vi "_Copy 1.vi"(0 "XRef":T5, 1 "State In":T1) -> (14 "Reply":T3, 15 "Fatal Error Out":T2, 16 "State Out":T1)   [LabVIEW 2014, in "JKISM++ DebugTool.xnode"]
uses:
  JKISM++ DebugTool.xnode
  <vilib>/XNodeSupport/XNodeXNodeRef.ctl
  _State 1.ctl
  <vilib>/XNodeSupport/XNodeStringArray.ctl
  <vilib>/XNodeSupport/XNodeString.ctl
  <vilib>/XNodeSupport/XNodeErrorCluster.ctl
  <vilib>/XNodeSupport/NI_XNodeSupport.lvlib
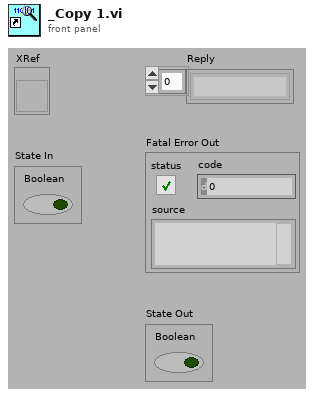
[diagram p1: front panel]
types:
  T1 = typedef "JKISM++ DebugTool.xnode/_State 1.ctl" = cluster{"Boolean":bool}
  T2 = typedef "NI_XNodeSupport.lvlib/XNodeErrorCluster.ctl" = errorcluster
  T3 = typedef "NI_XNodeSupport.lvlib/XNodeStringArray.ctl" = T4[]
  T4 = typedef "NI_XNodeSupport.lvlib/XNodeString.ctl" = string
  T5 = typedef "NI_XNodeSupport.lvlib/XNodeXNodeRef.ctl" = refnum<vi>
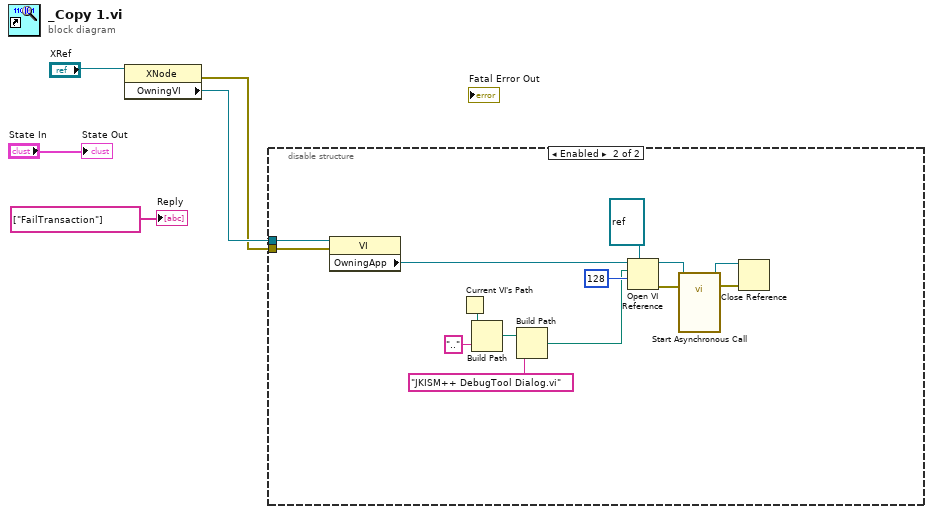
[diagram p0: block diagram]
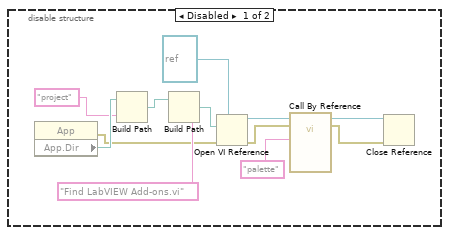
[diagram p2: hidden frame]
diagram:
  n1 = property class="XNode"(reference="XRef") -> (error out=w1:errorcluster, "OwningVI"=w2:refnum<vi>)  [unwired: 1 in, 1 out]
  n2 = disable-structure shown="Enabled" {
    disable-tunnel: w2 -> [_ w23]
    disable-tunnel: w1 -> [_ w18]
    frame Disabled {
      n3 = property class="App"() -> (error out=w12:errorcluster, "App.Dir"=w17:path)  [unwired: 2 in, 1 out]
      n4 = Build Path(base path=w17, name or relative path="project") -> (appended path=w15:path)
      n5 = Build Path(base path=w15, name or relative path="Find LabVIEW Add-ons.vi") -> (appended path=w13:path)
      n6 = Open VI Reference(type specifier VI Refnum (for type only)=refnum<vi> refnum ("reference"), vi path=w13, error in (no error)=w12) -> (vi reference=w10:refnum<vi>, error out=w7:errorcluster)  [unwired: 3 in]
      n7 = call-by-ref "?"(reference=w10, error in=w7, "Source"="palette") -> (reference out=w6:refnum<vi>, error out=w8:errorcluster)  [unwired: 11 in]
      n8 = Close Reference(reference=w6, error in (no error)=w8) -> ()  [unwired: 1 out]
    }
    frame Enabled {
      n9 = property class="VI"(reference=w23, error in=w18) -> ("OwningApp"=w22:refnum<vi>)  [unwired: 2 out]
      n10 = Current VI's Path() -> (path=w20:path)
      n11 = Build Path(base path=w20, name or relative path="..") -> (appended path=w19:path)
      n12 = Build Path(base path=w19, name or relative path="JKISM++ DebugTool Dialog.vi") -> (appended path=w25:path)
      n13 = Open VI Reference(type specifier VI Refnum (for type only)=refnum<vi> refnum, application reference (local)=w22, vi path=w25, options=128) -> (vi reference=w27:refnum<vi>, error out=w26:errorcluster)  [unwired: 2 in]
      n14 = call-by-ref "Start Asynchronous Call"(reference=w27, error in=w26) -> (reference out=w29:refnum<vi>, error out=w28:errorcluster)  [unwired: 12 in]
      n15 = Close Reference(reference=w29, error in (no error)=w28) -> ()  [unwired: 1 out]
    }
  }
  "Reply" <- T3 ["FailTransaction"] ("Reply")
  "State Out" <- "State In"
